vi "S4GUI_002.vi"(7 "Tab ObsEng":enum32{"Obs", "CCD modes", "Eng"}(tab)) -> ()   [LabVIEW 2018] (continued)
                      frame 0 {
                      }
                      frame 1 {
                      }
                      frame 2 {
                      }
                      frame 3 {
                        n288 = case shown="True" w572 {
                          tunnel: [cluster{u32, u32}[] [{7563008, 7563008}, {7563008, 7563008}] ("Colors [4]") cluster{u32, u32}[] [{16318208, 16318208}, {16318208, 16318208}] ("Colors [4]")] -> w571
                          frame False {
                          }
                          frame True {
                          }
                        }
                        n289 = Not(x=w572) -> (.not. x?=w573:bool)
                      }
                    }
                    "WPSEL Status" <- w554
                    "Waveplate" <- w554
                    n290 = property on="Waveplate" class="Bool (strict)"("Colors [4]"=w555, "BoolText.Text"=w551) -> ()  [unwired: 2 in, 2 out]
                    n291 = property on="WPSEL Status" class="Bool (strict)"("Colors [4]"=w555) -> ()  [unwired: 2 in, 2 out]
                  }
                  frame #1 {
                    # "WPROT"
                    n292 = Unbundle By Name(w579) -> ("WPROT State"=w578:i32)
                    n293 = case shown="2" w578 {
                      tunnel: [cluster{u32, u32}[] [{9868950, 9868950}, {9868950, 9868950}] ("Colors [4]") cluster{u32, u32}[] [{9868950, 9868950}, {9868950, 9868950}] ("Colors [4]") cluster{u32, u32}[] [{16318208, 16318208}, {16318208, 16318208}] ("Colors [4]") cluster{u32, u32}[] [{6618880, 6618880}, {6618880, 6618880}] ("Colors [4]") cluster{u32, u32}[] [{16318208, 16318208}, {16318208, 16318208}] ("Colors [4]")] -> w577
                      tunnel: [FALSE ("WPROT Status") FALSE ("WPROT Status") TRUE ("WPROT Status") FALSE ("WPROT Status") TRUE ("WPROT Status")] -> w576
                      frame Default {
                      }
                      frame 0 {
                      }
                      frame 1 {
                      }
                      frame 2 {
                      }
                      frame 3 {
                      }
                    }
                    "WPROT Status" <- w576
                    n294 = property on="WPROT Status" class="Bool (strict)"("Colors [4]"=w577) -> ()  [unwired: 2 in, 2 out]
                  }
                  frame #2 {
                    # "CALW"
                    n295 = Unbundle By Name(w597) -> ("CALW State"=w596:i32)
                    n296 = Unbundle By Name(w595) -> ("CALW posname"=w594:string)
                    n297 = local read "CALW Status"() -> (w590:bool)
                    n298 = case shown="3" w596 {
                      tunnel: [cluster{u32, u32}[] [{9868950, 9868950}, {9868950, 9868950}] ("Colors [4]") cluster{u32, u32}[] [{9868950, 9868950}, {9868950, 9868950}] ("Colors [4]") cluster{u32, u32}[] [{16318208, 16318208}, {16318208, 16318208}] ("Colors [4]") cluster{u32, u32}[] [{6618880, 6618880}, {6618880, 6618880}] ("Colors [4]") w617] -> w591
                      tunnel: [FALSE ("WPROT Status") FALSE ("WPROT Status") TRUE ("WPROT Status") FALSE ("WPROT Status") w619] -> w593
                      tunnel: w594 -> [_ _ _ w608 _]
                      tunnel: ["" "" "" w607 ""] -> w592
                      tunnel: w590 -> [_ _ _ _ w618]
                      frame Default {
                      }
                      frame 0 {
                      }
                      frame 1 {
                      }
                      frame 2 {
                        n299 = case shown="\"SHUTTER\"" w608 {
                          tunnel: ["" "DEPOL" "POL" "OFF" "PIN" "SHT"] -> w607
                          frame Default {
                          }
                          frame "DEPOLARIZER" {
                          }
                          frame "POLARIZER" {
                          }
                          frame "OFF" {
                          }
                          frame "PINHOLE" {
                          }
                          frame "SHUTTER" {
                          }
                        }
                      }
                      frame 3 {
                        n300 = case shown="False" w618 {
                          tunnel: [cluster{u32, u32}[] [{7563008, 7563008}, {7563008, 7563008}] ("Colors [4]") cluster{u32, u32}[] [{16318208, 16318208}, {16318208, 16318208}] ("Colors [4]")] -> w617
                          frame False {
                          }
                          frame True {
                          }
                        }
                        n301 = Not(x=w618) -> (.not. x?=w619:bool)
                      }
                    }
                    "CALW Status" <- w593
                    "PCS" <- w593
                    n302 = property on="CALW Status" class="Bool (strict)"("Colors [4]"=w591) -> ()  [unwired: 2 in, 2 out]
                    n303 = property on="PCS" class="Bool (strict)"("Colors [4]"=w591, "BoolText.Text"=w592) -> ()  [unwired: 2 in, 2 out]
                  }
                  frame #3 {
                    # "ASEL"
                    n304 = Unbundle By Name(w631) -> ("ASEL State"=w630:i32)
                    n305 = Unbundle By Name(w627) -> ("ASEL posname"=w624:string)
                    n306 = local read "ASEL Status"() -> (w625:bool)
                    n307 = case shown="Default" w624 {
                      selector: w624 -> [w632 _ _]
                      tunnel: [w632 "OFF" ("y") "ON" ("y")] -> w623
                      frame Default {
                      }
                      frame "OFF" {
                      }
                      frame "ON" {
                      }
                    }
                    n308 = case shown="3" w630 {
                      tunnel: [cluster{u32, u32}[] [{9868950, 9868950}, {9868950, 9868950}] ("Colors [4]") cluster{u32, u32}[] [{9868950, 9868950}, {9868950, 9868950}] ("Colors [4]") cluster{u32, u32}[] [{16318208, 16318208}, {16318208, 16318208}] ("Colors [4]") cluster{u32, u32}[] [{6618880, 6618880}, {6618880, 6618880}] ("Colors [4]") w650] -> w628
                      tunnel: [FALSE ("WPROT Status") FALSE ("WPROT Status") TRUE FALSE ("WPROT Status") w649] -> w629
                      tunnel: w623 -> [_ _ _ w645 _]
                      tunnel: ["" ("y") "" ("y") "" ("y") w645 "" ("y")] -> w626
                      tunnel: w625 -> [_ _ _ _ w647]
                      frame Default {
                      }
                      frame 0 {
                      }
                      frame 1 {
                      }
                      frame 2 {
                      }
                      frame 3 {
                        n309 = case shown="True" w647 {
                          tunnel: [cluster{u32, u32}[] [{7563008, 7563008}, {7563008, 7563008}] ("Colors [4]") cluster{u32, u32}[] [{16318208, 16318208}, {16318208, 16318208}] ("Colors [4]")] -> w650
                          frame False {
                          }
                          frame True {
                          }
                        }
                        n310 = Not(x=w647) -> (.not. x?=w649:bool)
                      }
                    }
                    "ASEL Status" <- w629
                    "Analyzer" <- w629
                    n311 = property on="Analyzer" class="Bool (strict)"("Colors [4]"=w628, "BoolText.Text"=w626) -> ()  [unwired: 2 in, 2 out]
                    n312 = property on="ASEL Status" class="Bool (strict)"("Colors [4]"=w628) -> ()  [unwired: 2 in, 2 out]
                  }
                  frame #4 {
                    # "GMIR & GFOC"
                    n313 = Unbundle By Name(w660) -> ("GMIR State"=w659:i32, "GFOC State"=w656:i32)
                    n314 = case shown="Default" w659 {
                      tunnel: [cluster{u32, u32}[] [{9868950, 9868950}, {9868950, 9868950}] ("Colors [4]") cluster{u32, u32}[] [{9868950, 9868950}, {9868950, 9868950}] ("Colors [4]") cluster{u32, u32}[] [{16318208, 16318208}, {16318208, 16318208}] ("Colors [4]") cluster{u32, u32}[] [{6618880, 6618880}, {6618880, 6618880}] ("Colors [4]") cluster{u32, u32}[] [{16318208, 16318208}, {16318208, 16318208}] ("Colors [4]")] -> w658
                      tunnel: [FALSE ("WPROT Status") FALSE ("WPROT Status") TRUE ("WPROT Status") FALSE ("WPROT Status") TRUE ("WPROT Status")] -> w655
                      frame Default {
                      }
                      frame 0 {
                      }
                      frame 1 {
                      }
                      frame 2 {
                      }
                      frame 3 {
                      }
                    }
                    "GMIR Status" <- w655
                    n315 = property on="GMIR Status" class="Bool (strict)"("Colors [4]"=w658) -> ()  [unwired: 2 in, 2 out]
                    n316 = case shown="Default" w656 {
                      tunnel: [cluster{u32, u32}[] [{9868950, 9868950}, {9868950, 9868950}] ("Colors [4]") cluster{u32, u32}[] [{9868950, 9868950}, {9868950, 9868950}] ("Colors [4]") cluster{u32, u32}[] [{16318208, 16318208}, {16318208, 16318208}] ("Colors [4]") cluster{u32, u32}[] [{6618880, 6618880}, {6618880, 6618880}] ("Colors [4]") cluster{u32, u32}[] [{16318208, 16318208}, {16318208, 16318208}] ("Colors [4]")] -> w657
                      tunnel: [FALSE ("WPROT Status") FALSE ("WPROT Status") TRUE ("WPROT Status") FALSE ("WPROT Status") TRUE ("WPROT Status")] -> w654
                      frame Default {
                      }
                      frame 0 {
                      }
                      frame 1 {
                      }
                      frame 2 {
                      }
                      frame 3 {
                      }
                    }
                    "GFOC Status" <- w654
                    n317 = Or(x=w655, y=w654) -> (x .or. y?=w653:bool)
                    n318 = property on="GFOC Status" class="Bool (strict)"("Colors [4]"=w657) -> ()  [unwired: 2 in, 2 out]
                    n319 = property on="GS led" class="Bool (strict)"("Blinking"=w653, "Value"=w653) -> ()  [unwired: 2 in, 2 out]
                  }
                }
              }
              frame #7 {
                n320 = Unbundle By Name(w683) -> ("Instrument Pos Names"=w682:T21)
                n321 = stacked-sequence {
                  tunnel: w682 -> [w685 w702 w727 w753]
                  tunnel: [_ _ _ w754] -> w681
                  frame #0 {
                    n322 = Unbundle By Name(w685) -> ("WPSEL posname"=w684:string)
                    n323 = case shown="\"L/2\", \"L/4\", \"OFF\"" w684 {
                      selector: w684 -> [_ w686]
                      frame "False", Default {
                      }
                      frame "L/2", "L/4", "OFF" {
                        n324 = First Call?() -> (First Call?: T/F=w687:bool)
                        n325 = case shown="True" w687 {
                          tunnel: w686 -> [_ w688]
                          frame False {
                          }
                          frame True {
                            n326 = case shown="\"OFF\"" w688 {
                              frame "False", Default {
                              }
                              frame "L/2" {
                                w689 = u16 1 items=["OFF", "Lambda/2", "Lambda/4"] ("Lambda Selector")
                                n327 = property on="Lambda Selector" class="Ring (strict)"(error in=errorcluster {"status"=FALSE, "code"=0, "source"=""} ("error in (no error)"), "Value"=w689) -> (error out=w691:errorcluster)  [unwired: 1 in, 1 out]
                                n328 = property on="Lambda Selector" class="Ring (strict)"(error in=w691, "RingText.Text"="Lambda/2" ("Boolean Text.Text")) -> ()  [unwired: 1 in, 2 out]
                              }
                              frame "L/4" {
                                w693 = u16 2 items=["OFF", "Lambda/2", "Lambda/4"] ("Lambda Selector")
                                n329 = property on="Lambda Selector" class="Ring (strict)"(error in=errorcluster {"status"=FALSE, "code"=0, "source"=""} ("error in (no error)"), "Value"=w693) -> (error out=w695:errorcluster)  [unwired: 1 in, 1 out]
                                n330 = property on="Lambda Selector" class="Ring (strict)"(error in=w695, "RingText.Text"="Lambda/4" ("Boolean Text.Text")) -> ()  [unwired: 1 in, 2 out]
                              }
                              frame "OFF" {
                                w698 = u16 0 items=["OFF", "Lambda/2", "Lambda/4"] ("Lambda Selector")
                                (unwired) "Select..." ("Boolean Text.Text")
                                n331 = property on="Lambda Selector" class="Ring (strict)"(error in=errorcluster {"status"=FALSE, "code"=0, "source"=""} ("error in (no error)"), "Value"=w698) -> (error out=w700:errorcluster)  [unwired: 1 in, 1 out]
                                n332 = property on="Lambda Selector" class="Ring (strict)"(error in=w700, "RingText.Text"="OFF" ("Boolean Text.Text")) -> ()  [unwired: 1 in, 2 out]
                              }
                            }
                          }
                        }
                      }
                    }
                  }
                  frame #1 {
                    n333 = Unbundle By Name(w702) -> ("CALW posname"=w701:string)
                    n334 = case shown="\"DEPOLARIZER\", \"OFF\", \"PINHOLE\", \"POLARIZER\", \"SHUTTER\"" w701 {
                      selector: w701 -> [_ w703]
                      frame "False", Default {
                      }
                      frame "DEPOLARIZER", "OFF", "PINHOLE", "POLARIZER", "SHUTTER" {
                        n335 = First Call?() -> (First Call?: T/F=w704:bool)
                        n336 = case shown="True" w704 {
                          tunnel: w703 -> [_ w705]
                          frame False {
                          }
                          frame True {
                            n337 = case shown="\"OFF\"" w705 {
                              frame "False", Default {
                              }
                              frame "POLARIZER" {
                                w706 = u16 1 items=["OFF", "POLARIZER", "PINHOLE", "SHUTTER", "DEPOLARIZER"] ("Calibrator Selector")
                                n338 = property on="Calibrator Selector" class="Ring (strict)"(error in=errorcluster {"status"=FALSE, "code"=0, "source"=""} ("error in (no error)"), "Value"=w706) -> (error out=w708:errorcluster)  [unwired: 1 in, 1 out]
                                n339 = property on="Calibrator Selector" class="Ring (strict)"(error in=w708, "RingText.Text"="POLARIZER" ("Boolean Text.Text")) -> ()  [unwired: 1 in, 2 out]
                              }
                              frame "DEPOLARIZER" {
                                w710 = u16 4 items=["OFF", "POLARIZER", "PINHOLE", "SHUTTER", "DEPOLARIZER"] ("Calibrator Selector")
                                n340 = property on="Calibrator Selector" class="Ring (strict)"(error in=errorcluster {"status"=FALSE, "code"=0, "source"=""} ("error in (no error)"), "Value"=w710) -> (error out=w712:errorcluster)  [unwired: 1 in, 1 out]
                                n341 = property on="Calibrator Selector" class="Ring (strict)"(error in=w712, "RingText.Text"="DEPOLARIZER" ("Boolean Text.Text")) -> ()  [unwired: 1 in, 2 out]
                              }
                              frame "PINHOLE" {
                                w714 = u16 2 items=["OFF", "POLARIZER", "PINHOLE", "SHUTTER", "DEPOLARIZER"] ("Calibrator Selector")
                                n342 = property on="Calibrator Selector" class="Ring (strict)"(error in=errorcluster {"status"=FALSE, "code"=0, "source"=""} ("error in (no error)"), "Value"=w714) -> (error out=w716:errorcluster)  [unwired: 1 in, 1 out]
                                n343 = property on="Calibrator Selector" class="Ring (strict)"(error in=w716, "RingText.Text"="PINHOLE" ("Boolean Text.Text")) -> ()  [unwired: 1 in, 2 out]
                              }
                              frame "SHUTTER" {
                                w718 = u16 3 items=["OFF", "POLARIZER", "PINHOLE", "SHUTTER", "DEPOLARIZER"] ("Calibrator Selector")
                                n344 = property on="Calibrator Selector" class="Ring (strict)"(error in=errorcluster {"status"=FALSE, "code"=0, "source"=""} ("error in (no error)"), "Value"=w718) -> (error out=w720:errorcluster)  [unwired: 1 in, 1 out]
                                n345 = property on="Calibrator Selector" class="Ring (strict)"(error in=w720, "RingText.Text"="SHUTTER" ("Boolean Text.Text")) -> ()  [unwired: 1 in, 2 out]
                              }
                              frame "OFF" {
                                w722 = u16 0 items=["OFF", "POLARIZER", "PINHOLE", "SHUTTER", "DEPOLARIZER"] ("Calibrator Selector")
                                n346 = property on="Calibrator Selector" class="Ring (strict)"(error in=errorcluster {"status"=FALSE, "code"=0, "source"=""} ("error in (no error)"), "Value"=w722) -> (error out=w724:errorcluster)  [unwired: 1 in, 1 out]
                                n347 = property on="Calibrator Selector" class="Ring (strict)"(error in=w724, "RingText.Text"="OFF" ("Boolean Text.Text")) -> ()  [unwired: 1 in, 2 out]
                              }
                            }
                          }
                        }
                      }
                    }
                  }
                  frame #2 {
                    n348 = Unbundle By Name(w727) -> ("WPROT posname"=w726:string)
                    "Name" <- w726
                    n349 = stacked-sequence {
                      tunnel: w726 -> [_ w729]
                      frame #0 {
                        w728 = FALSE
                        "ledP0" <- w728
                        "ledP1" <- w728
                        "ledP2" <- w728
                        "ledP3" <- w728
                        "ledP4" <- w728
                        "ledP5" <- w728
                        "ledP6" <- w728
                        "ledP7" <- w728
                        "ledP8" <- w728
                        "ledP9" <- w728
                        "ledP10" <- w728
                        "ledP11" <- w728
                        "ledP12" <- w728
                        "ledP13" <- w728
                        "ledP14" <- w728
                        "ledP15" <- w728
                      }
                      frame #1 {
                        n350 = case shown="\"WP3\"" w729 {
                          frame Default {
                          }
                          frame "WP1" {
                            n351 = local write "ledP0"(TRUE ("ledP0")) -> ()
                          }
                          frame "WP2" {
                            n352 = local write "ledP1"(TRUE ("ledP0")) -> ()
                          }
                          frame "WP3" {
                            n353 = local write "ledP2"(TRUE ("ledP0")) -> ()
                          }
                          frame "WP4" {
                            n354 = local write "ledP3"(TRUE ("ledP0")) -> ()
                          }
                          frame "WP5" {
                            n355 = local write "ledP4"(TRUE ("ledP0")) -> ()
                          }
                          frame "WP6" {
                            n356 = local write "ledP5"(TRUE ("ledP0")) -> ()
                          }
                          frame "WP7" {
                            n357 = local write "ledP6"(TRUE ("ledP0")) -> ()
                          }
                          frame "WP8" {
                            n358 = local write "ledP7"(TRUE ("ledP0")) -> ()
                          }
                          frame "WP9" {
                            n359 = local write "ledP8"(TRUE ("ledP0")) -> ()
                          }
                          frame "WP10" {
                            n360 = local write "ledP9"(TRUE ("ledP0")) -> ()
                          }
                          frame "WP11" {
                            n361 = local write "ledP10"(TRUE ("ledP0")) -> ()
                          }
                          frame "WP12" {
                            n362 = local write "ledP11"(TRUE ("ledP0")) -> ()
                          }
                          frame "WP13" {
                            n363 = local write "ledP12"(TRUE ("ledP0")) -> ()
                          }
                          frame "WP14" {
                            n364 = local write "ledP13"(TRUE ("ledP0")) -> ()
                          }
                          frame "WP15" {
                            n365 = local write "ledP14"(TRUE ("ledP0")) -> ()
                          }
                          frame "WP16" {
                            n366 = local write "ledP15"(TRUE ("ledP0")) -> ()
                          }
                        }
                      }
                    }
                  }
                  frame #3 {
                    w757 = "OFF" ("Boolean Text.Text")
                    # "Polarimetria:   ASEL = ON  &   (WPSEL =L/2 or L/4)\n\nFotometria:    ASEL=OFF & WPSEL = OFF & CALW = OFF"
                    n367 = Unbundle By Name(w753) -> ("ASEL posname"=w748:string, "WPSEL posname"=w750:string, "CALW posname"=w749:string)
                    n368 = Unbundle By Name(w753) -> ("WPSEL posname"=w760:string, "CALW posname"=w761:string, "ASEL posname"=w755:string)
                    n369 = Equal?(x=w748, y="ON" ("Boolean Text.Text")) -> (x = y?=w751:bool)
                    n370 = case shown="True" w751 {
                      tunnel: w750 -> [w770 w779]
                      tunnel: w749 -> [w769 w773]
                      tunnel: w748 -> [w766 _]
                      tunnel: [FALSE ("Polarimetric Mode") w774] -> w747
                      tunnel: [w762 FALSE ("Photometric Mode")] -> w746
                      frame False {
                        w765 = "OFF" ("Boolean Text.Text")
                        n371 = Equal?(x=w766, y=w765) -> (x = y?=w764:bool)
                        n372 = Equal?(x=w769, y=w765) -> (x = y?=w767:bool)
                        n373 = Equal?(x=w770, y=w765) -> (x = y?=w768:bool)
                        n374 = Compound Arithmetic op=AND(w764, w768, w767) -> (w762:bool)
                      }
                      frame True {
                        n375 = Equal?(x="L/2" ("Boolean Text.Text"), y=w779) -> (x = y?=w780:bool)
                        n376 = Equal?(x="L/4" ("Boolean Text.Text"), y=w779) -> (x = y?=w777:bool)
                        n377 = Not Equal?(x="SHUTTER", y=w773) -> (x != y?=w771:bool)
                        n378 = Or(x=w780, y=w777) -> (x .or. y?=w775:bool)
                        n379 = And(x=w775, y=w771) -> (x .and. y?=w774:bool)
                      }
                    }
                    "Polarimetric Mode" <- w747
                    "Photometric Mode" <- w746
                    n380 = Equal?(x=w757, y=w760) -> (x = y?=w758:bool)
                    n381 = Equal?(x=w757, y=w761) -> (x = y?=w759:bool)
                    n382 = Equal?(x=w757, y=w755) -> (x = y?=w756:bool)
                    n383 = Compound Arithmetic op=AND(w758, w759, w756) -> (invert w754:bool)
                  }
                }
              }
              frame #8 {
                n384 = Unbundle By Name(w786) -> ("ChannelA_Status"=w785:T22, "ChannelB_Status"=w784:T22, "ChannelC_Status"=w782:T22, "ChannelD_Status"=w783:T22)
                n385 = stacked-sequence {
                  tunnel: w785 -> [w874 w930 w982 w1059 _ _ _]
                  tunnel: w784 -> [w873 w928 w981 _ w1080 _ _]
                  tunnel: w783 -> [w871 w925 w979 _ _ _ w1122]
                  tunnel: w782 -> [w872 w926 w980 _ _ w1101 _]
                  frame #0 {
                    n386 = Unbundle By Name(w871) -> ("connection"=w851:bool, "FT"=w833:bool, "Current exp"=w810:dbl, "Cooler ON/OFF"=w865:i16, "Currently temperature"=w862:i16, "Temperature Status"=w859:string, "target  temp"=w795:i16)
                    "Exposure Time ch4" <- w810
                    n387 = Unbundle By Name(w873) -> ("connection"=w853:bool, "FT"=w837:bool, "Current exp"=w821:dbl, "Cooler ON/OFF"=w867:i16, "Currently temperature"=w864:i16, "Temperature Status"=w861:string, "target  temp"=w799:i16)
                    "Exposure Time ch2" <- w821
                    n388 = Unbundle By Name(w874) -> ("connection"=w854:bool, "FT"=w838:bool, "Current exp"=w830:dbl, "Cooler ON/OFF"=w870:i16, "Currently temperature"=w868:i16, "Temperature Status"=w869:string, "target  temp"=w807:i16)
                    "Exposure Time ch1" <- w830
                    n389 = Unbundle By Name(w872) -> ("connection"=w852:bool, "FT"=w835:bool, "Current exp"=w811:dbl, "Cooler ON/OFF"=w866:i16, "Currently temperature"=w863:i16, "Temperature Status"=w860:string, "target  temp"=w796:i16)
                    "Exposure Time ch3" <- w811
                    n390 = Number To Decimal String(number=w795) -> (decimal integer string=→"Target Temp 4":string)  [unwired: 1 in]
                    n391 = Number To Decimal String(number=w796) -> (decimal integer string=→"Target Temp 3":string)  [unwired: 1 in]
                    n392 = Number To Decimal String(number=w799) -> (decimal integer string=→"Target Temp 2":string)  [unwired: 1 in]
                    n393 = Not Equal To 0?(x=w865) -> (x != 0?=w856:bool)
                    n394 = First Call?() -> (First Call?: T/F=w848:bool)
                    n395 = First Call?() -> (First Call?: T/F=w850:bool)
                    n396 = First Call?() -> (First Call?: T/F=w847:bool)
                    n397 = Not Equal To 0?(x=w866) -> (x != 0?=w855:bool)
                    n398 = First Call?() -> (First Call?: T/F=w849:bool)
                    n399 = Number To Decimal String(number=w807) -> (decimal integer string=→"Target Temp 1":string)  [unwired: 1 in]
                    n400 = Number To Fractional String(use system decimal point (T)=FALSE, number=w830, precision (6)=i16 2) -> (F-format string=w827:string)  [unwired: 1 in]
                    n401 = case shown="True" w848 {
                      tunnel: w796 -> [_ w876]
                      frame False {
                      }
                      frame True {
                        n402 = property on="Target Temp 3" class="DigNum (strict)"("Value"=w876) -> ()  [unwired: 2 in, 2 out]
                      }
                    }
                    n403 = case shown="True" w850 {
                      tunnel: w807 -> [_ w878]
                      frame False {
                      }
                      frame True {
                        n404 = property on="Target Temp 1" class="DigNum (strict)"("Value"=w878) -> ()  [unwired: 2 in, 2 out]
                      }
                    }
                    n405 = Number To Fractional String(use system decimal point (T)=FALSE, number=w821, precision (6)=i16 2) -> (F-format string=w822:string)  [unwired: 1 in]
                    n406 = case shown="True" w847 {
                      tunnel: w795 -> [_ w875]
                      frame False {
                      }
                      frame True {
                        n407 = property on="Target Temp 4" class="DigNum (strict)"("Value"=w875) -> ()  [unwired: 2 in, 2 out]
                      }
                    }
                    n408 = Concatenate Strings("Exposure Time ", w827) -> (w826:string)
                    n409 = Number To Fractional String(use system decimal point (T)=FALSE, number=w811, precision (6)=i16 2) -> (F-format string=w812:string)  [unwired: 1 in]
                    n410 = Number To Fractional String(use system decimal point (T)=FALSE, number=w810, precision (6)=i16 2) -> (F-format string=w816:string)  [unwired: 1 in]
                    n411 = Concatenate Strings("Exposure Time ", w822) -> (w820:string)
                    n412 = case shown="True" w849 {
                      tunnel: w799 -> [_ w877]
                      frame False {
                      }
                      frame True {
                        n413 = property on="Target Temp 2" class="DigNum (strict)"("Value"=w877) -> ()  [unwired: 2 in, 2 out]
                      }
                    }
                    n414 = Concatenate Strings("Exposure Time ", w812) -> (w808:string)
                    n415 = Concatenate Strings("Exposure Time ", w816) -> (w809:string)
                    n416 = property on="Exposure Time ch1" class="Slide (strict)"("Caption.Text"=w826) -> ()  [unwired: 2 in, 2 out]
                    n417 = property on="Exposure Time ch2" class="Slide (strict)"("Caption.Text"=w820) -> ()  [unwired: 2 in, 2 out]
                    n418 = property on="Exposure Time ch3" class="Slide (strict)"("Caption.Text"=w808) -> ()  [unwired: 2 in, 2 out]
                    n419 = property on="Exposure Time ch4" class="Slide (strict)"("Caption.Text"=w809) -> ()  [unwired: 2 in, 2 out]
                    n420 = Not Equal To 0?(x=w870) -> (x != 0?=w857:bool)
                    n421 = Not Equal To 0?(x=w867) -> (x != 0?=w858:bool)
                    n422 = case shown="True" w854 {
                      tunnel: w869 -> [_ w909]
                      tunnel: w868 -> [_ w910]
                      tunnel: w857 -> [_ w907]
                      tunnel: [FALSE w907] -> w846
                      tunnel: [i16 0 ("Currently temperature") w910] -> w804
                      tunnel: ["" ("Temperature Status") w909] -> w845
                      tunnel: [FALSE w908] -> w839
                      tunnel: w838 -> [_ w908]
                      frame False {
                      }
                      frame True {
                      }
                    }
                    "Cooler status 1" <- w846
                    "Curr Temp 1" <- w804
                    "Temp Status 1" <- w845
                    "Panel Temp" <- w804
                    "Panel cooler 1" <- w846
                    "FT1" <- w839
                    n423 = case shown="False" w853 {
                      tunnel: w864 -> [_ w901]
                      tunnel: w861 -> [_ w900]
                      tunnel: w858 -> [_ w902]
                      tunnel: [FALSE w902] -> w844
                      tunnel: [i16 0 ("Currently temperature") w901] -> w800
                      tunnel: ["" ("Temperature Status") w900] -> w843
                      tunnel: w837 -> [_ w899]
                      tunnel: [FALSE ("FT") w899] -> w836
                      frame False {
                      }
                      frame True {
                      }
                    }
                    "Panel Temp 2" <- w800
                    "Curr Temp 2" <- w800
                    "Cooler status 2" <- w844
                    "Panel cooler 2" <- w844
                    "Temp Status 2" <- w843
                    "FT2" <- w836
                    n424 = case shown="True" w851 {
                      tunnel: w862 -> [_ w885]
                      tunnel: w859 -> [_ w884]
                      tunnel: w856 -> [_ w886]
                      tunnel: [FALSE w886] -> w841
                      tunnel: [i16 0 ("Currently temperature") w885] -> w788
                      tunnel: ["" ("Temperature Status") w884] -> w840
                      tunnel: w833 -> [_ w883]
                      tunnel: [FALSE ("FT") w883] -> w832
                      frame False {
                      }
                      frame True {
                      }
                    }
                    "Cooler status 4" <- w841
                    "Panel Temp 4" <- w788
                    "Curr Temp 4" <- w788
                    "Temp Status 4" <- w840
                    "Panel cooler 4" <- w841
                    "FT4" <- w832
                    n425 = case shown="True" w852 {
                      tunnel: w863 -> [_ w893]
                      tunnel: w860 -> [_ w892]
                      tunnel: w855 -> [_ w894]
                      tunnel: [FALSE w894] -> w842
                      tunnel: [i16 0 ("Currently temperature") w893] -> w789
                      tunnel: ["" ("Temperature Status") w892] -> w787
                      tunnel: w835 -> [_ w891]
                      tunnel: [FALSE ("FT") w891] -> w834
                      frame False {
                      }
                      frame True {
                      }
                    }
                    "Cooler status 3" <- w842
                    "Panel Temp 3" <- w789
                    "Curr Temp 3" <- w789
                    "Panel cooler 3" <- w842
                    "FT3" <- w834
                    "Temp Status 3" <- w787
                    n426 = Number To Decimal String(number=w800) -> (decimal integer string=w801:string)  [unwired: 1 in]
                    n427 = Number To Decimal String(number=w804) -> (decimal integer string=w805:string)  [unwired: 1 in]
                    n428 = property on="Panel cooler 2" class="Bool (strict)"("BoolText.Text"=w801, "BoolText.Justify"=enum16{"Left", "Center", "Right"}."Right" ("Boolean Text.Justification")) -> ()  [unwired: 2 in, 2 out]
                    n429 = property on="Panel cooler 1" class="Bool (strict)"("BoolText.Text"=w805, "BoolText.Justify"=enum16{"Left", "Center", "Right"}."Right" ("Boolean Text.Justification")) -> ()  [unwired: 2 in, 2 out]
                    n430 = Number To Decimal String(number=w789) -> (decimal integer string=w793:string)  [unwired: 1 in]
                    n431 = Number To Decimal String(number=w788) -> (decimal integer string=w790:string)  [unwired: 1 in]
                    n432 = property on="Panel cooler 3" class="Bool (strict)"("BoolText.Text"=w793, "BoolText.Justify"=enum16{"Left", "Center", "Right"}."Right" ("Boolean Text.Justification")) -> ()  [unwired: 2 in, 2 out]
                    n433 = property on="Panel cooler 4" class="Bool (strict)"("BoolText.Text"=w790, "BoolText.Justify"=enum16{"Left", "Center", "Right"}."Right" ("Boolean Text.Justification")) -> ()  [unwired: 2 in, 2 out]
                  }
                  frame #1 {
                    n434 = Unbundle By Name(w925) -> ("LastFileImage"=→"Last Image ch4":string, "Temperature Status"=w913:string)
                    n435 = Unbundle By Name(w926) -> ("LastFileImage"=→"Last Image ch3":string, "Temperature Status"=w914:string)
                    n436 = Unbundle By Name(w928) -> ("LastFileImage"=→"Last Image ch2":string, "Temperature Status"=w917:string)
                    n437 = Unbundle By Name(w930) -> ("LastFileImage"=→"Last Image ch1":string, "Temperature Status"=w922:string)
                    n438 = case shown="Default" w922 {
                      tunnel: [cluster{u32, u32}[] [{6124107, 6124107}, {6124107, 6124107}] ("Colors [4]") cluster{u32, u32}[] [{6618880, 6618880}, {6618880, 6618880}] ("Colors [4]") cluster{u32, u32}[] [{16318208, 16318208}, {16318208, 16318208}] ("Colors [4]") cluster{u32, u32}[] [{8554752, 8554752}, {8554752, 8554752}] ("Colors [4]")] -> w921
                      tunnel: [FALSE FALSE FALSE TRUE] -> w920
                      frame Default {
                      }
                      frame "TEMPERATURE_STABILIZED" {
                      }
                      frame "TEMPERATURE_NOT_STABILIZED" {
                      }
                      frame "TEMPERATURE_NOT_REACHED" {
                      }
                    }
                    n439 = case shown="\"TEMPERATURE_NOT_REACHED\"" w917 {
                      tunnel: [cluster{u32, u32}[] [{6124107, 6124107}, {6124107, 6124107}] ("Colors [4]") cluster{u32, u32}[] [{6618880, 6618880}, {6618880, 6618880}] ("Colors [4]") cluster{u32, u32}[] [{16318208, 16318208}, {16318208, 16318208}] ("Colors [4]") cluster{u32, u32}[] [{8554752, 8554752}, {8554752, 8554752}] ("Colors [4]")] -> w919
                      tunnel: [FALSE FALSE FALSE TRUE] -> w918
                      frame Default {
                      }
                      frame "TEMPERATURE_STABILIZED" {
                      }
                      frame "TEMPERATURE_NOT_STABILIZED" {
                      }
                      frame "TEMPERATURE_NOT_REACHED" {
                      }
                    }
                    n440 = case shown="\"TEMPERATURE_NOT_REACHED\"" w914 {
                      tunnel: [cluster{u32, u32}[] [{6124107, 6124107}, {6124107, 6124107}] ("Colors [4]") cluster{u32, u32}[] [{6618880, 6618880}, {6618880, 6618880}] ("Colors [4]") cluster{u32, u32}[] [{16318208, 16318208}, {16318208, 16318208}] ("Colors [4]") cluster{u32, u32}[] [{8554752, 8554752}, {8554752, 8554752}] ("Colors [4]")] -> w916
                      tunnel: [FALSE FALSE FALSE TRUE] -> w915
                      frame Default {
                      }
                      frame "TEMPERATURE_STABILIZED" {
                      }
                      frame "TEMPERATURE_NOT_STABILIZED" {
                      }
                      frame "TEMPERATURE_NOT_REACHED" {
                      }
                    }
                    n441 = case shown="\"TEMPERATURE_NOT_REACHED\"" w913 {
                      tunnel: [cluster{u32, u32}[] [{6124107, 6124107}, {6124107, 6124107}] ("Colors [4]") cluster{u32, u32}[] [{6618880, 6618880}, {6618880, 6618880}] ("Colors [4]") cluster{u32, u32}[] [{16318208, 16318208}, {16318208, 16318208}] ("Colors [4]") cluster{u32, u32}[] [{8554752, 8554752}, {8554752, 8554752}] ("Colors [4]")] -> w912
                      tunnel: [FALSE FALSE FALSE TRUE] -> w911
                      frame Default {
                      }
                      frame "TEMPERATURE_STABILIZED" {
                      }
                      frame "TEMPERATURE_NOT_STABILIZED" {
                      }
                      frame "TEMPERATURE_NOT_REACHED" {
                      }
                    }
                    n442 = property on="Cooler status 1" class="Bool (strict)"("Colors [4]"=w921, "Blinking"=w920) -> ()  [unwired: 2 in, 2 out]
                    n443 = property on="Panel cooler 1" class="Bool (strict)"("Colors [4]"=w921, "Blinking"=w920) -> ()  [unwired: 2 in, 2 out]
                    n444 = property on="Cooler status 4" class="Bool (strict)"("Colors [4]"=w912, "Blinking"=w911) -> ()  [unwired: 2 in, 2 out]
                    n445 = property on="Cooler status 3" class="Bool (strict)"("Colors [4]"=w916, "Blinking"=w915) -> ()  [unwired: 2 in, 2 out]
                    n446 = property on="Panel cooler 4" class="Bool (strict)"("Colors [4]"=w912, "Blinking"=w911) -> ()  [unwired: 2 in, 2 out]
                    n447 = property on="Cooler status 2" class="Bool (strict)"("Colors [4]"=w919, "Blinking"=w918) -> ()  [unwired: 2 in, 2 out]
                    n448 = property on="Panel cooler 3" class="Bool (strict)"("Colors [4]"=w916, "Blinking"=w915) -> ()  [unwired: 2 in, 2 out]
                    n449 = property on="Panel cooler 2" class="Bool (strict)"("Colors [4]"=w919, "Blinking"=w918) -> ()  [unwired: 2 in, 2 out]
                  }
                  frame #2 {
                    n450 = Unbundle By Name(w981) -> ("CamStatus"=w974:string, "connection"=w973:bool)
                    n451 = Unbundle By Name(w980) -> ("CamStatus"=w970:string, "connection"=w969:bool)
                    n452 = Unbundle By Name(w979) -> ("CamStatus"=w966:string, "connection"=w965:bool)
                    n453 = Unbundle By Name(w982) -> ("CamStatus"=w978:string, "connection"=w976:bool)
                    n454 = case shown="True" w973 {
                      tunnel: w974 -> [_ w1013]
                      tunnel: [u32 16739417 w1014] -> w971
                      tunnel: ["" ("CamStatus") w1013] -> w972
                      frame False {
                      }
                      frame True {
                        n455 = property on="Acq status string ch2" class="Str"() -> ("Text.BGColor"=w1015:u32)  [unwired: 2 in, 2 out]
                        n456 = case shown="\"\"" w1013 {
                          tunnel: [u32 16688641 w1020 u32 13882323 u32 13882323] -> w1014
                          tunnel: w1015 -> [_ w1019 _ _]
                          frame Default {
                            # "WAITING_EXPOSE_COMMAND"
                          }
                          frame "ACTIVE" {
                            n457 = Equal?(x=w1019, y=u32 16776002) -> (x = y?=w1018:bool)
                            n458 = case shown="False" w1018 {
                              tunnel: [u32 16776002 u32 16449369] -> w1020
                              frame False {
                              }
                              frame True {
                              }
                            }
                          }
                          frame "IDLE" {
                          }
                          frame "" {
                            # "sem resposta do ACS"
                          }
                        }
                      }
                    }
                    "Acq status string ch2" <- w972
                    n459 = case shown="True" w965 {
                      tunnel: w966 -> [_ w985]
                      tunnel: [u32 16739417 w986] -> w963
                      tunnel: ["" ("CamStatus") w985] -> w964
                      frame False {
                      }
                      frame True {
                        n460 = property on="Acq status string ch4" class="Str"() -> ("Text.BGColor"=w987:u32)  [unwired: 2 in, 2 out]
                        n461 = case shown="\"IDLE\"" w985 {
                          tunnel: [u32 16688641 w992 u32 13882323 u32 13882323] -> w986
                          tunnel: w987 -> [_ w991 _ _]
                          frame Default {
                            # "WAITING_EXPOSE_COMMAND"
                          }
                          frame "ACTIVE" {
                            n462 = Equal?(x=w991, y=u32 16776002) -> (x = y?=w990:bool)
                            n463 = case shown="False" w990 {
                              tunnel: [u32 16776002 u32 16449369] -> w992
                              frame False {
                              }
                              frame True {
                              }
                            }
                          }
                          frame "IDLE" {
                          }
                          frame "" {
                            # "sem resposta do ACS"
                          }
                        }
                      }
                    }
                    "Acq status string ch4" <- w964
                    n464 = case shown="True" w969 {
                      tunnel: w970 -> [_ w999]
                      tunnel: [u32 16739417 w1000] -> w967
                      tunnel: ["" ("CamStatus") w999] -> w968
                      frame False {
                      }
                      frame True {
                        n465 = property on="Acq status string ch3" class="Str"() -> ("Text.BGColor"=w1001:u32)  [unwired: 2 in, 2 out]
                        n466 = case shown="\"\"" w999 {
                          tunnel: [u32 16688641 w1006 u32 13882323 u32 13882323] -> w1000
                          tunnel: w1001 -> [_ w1005 _ _]
                          frame Default {
                            # "WAITING_EXPOSE_COMMAND"
                          }
                          frame "ACTIVE" {
                            n467 = Equal?(x=w1005, y=u32 16776002) -> (x = y?=w1004:bool)
                            n468 = case shown="False" w1004 {
                              tunnel: [u32 16776002 u32 16449369] -> w1006
                              frame False {
                              }
                              frame True {
                              }
                            }
                          }
                          frame "IDLE" {
                          }
                          frame "" {
                            # "sem resposta do ACS"
                          }
                        }
                      }
                    }
                    "Acq status string ch3" <- w968
                    n469 = case shown="True" w976 {
                      tunnel: w978 -> [_ w1027]
                      tunnel: [u32 16739417 w1028] -> w977
                      tunnel: ["" ("CamStatus") w1027] -> w975
                      frame False {
                      }
                      frame True {
                        n470 = property on="Acq status string ch1" class="Str"() -> ("Text.BGColor"=w1029:u32)  [unwired: 2 in, 2 out]
                        n471 = case shown="\"\"" w1027 {
                          tunnel: [u32 16688641 w1034 u32 13882323 u32 13882323] -> w1028
                          tunnel: w1029 -> [_ w1033 _ _]
                          frame Default {
                            # "WAITING_EXPOSE_COMMAND"
                          }
                          frame "ACTIVE" {
                            n472 = Equal?(x=w1033, y=u32 16776002) -> (x = y?=w1032:bool)
                            n473 = case shown="False" w1032 {
                              tunnel: [u32 16776002 u32 16449369] -> w1034
                              frame False {
                              }
                              frame True {
                              }
                            }
                          }
                          frame "IDLE" {
                          }
                          frame "" {
                            # "sem resposta do ACS"
                          }
                        }
                      }
                    }
                    "Acq status string ch1" <- w975
                    n474 = property on="Acq status string ch2" class="Str"("Text.BGColor"=w971) -> ()  [unwired: 2 in, 2 out]
                    n475 = property on="Acq status string ch1" class="Str"("Text.BGColor"=w977) -> ()  [unwired: 2 in, 2 out]
                    n476 = property on="Acq status string ch3" class="Str"("Text.BGColor"=w967) -> ()  [unwired: 2 in, 2 out]
                    n477 = property on="Acq status string ch4" class="Str"("Text.BGColor"=w963) -> ()  [unwired: 2 in, 2 out]
                  }
                  frame #3 {
                    w1047 = cluster{u32, u32}[] [{16711680, 16711680}, {15400704, 15400704}, {16776722, 0}, {16776722, 0}]  # amarelo
                    w1046 = cluster{u32, u32}[] [{16711680, 16711680}, {6618880, 6618880}, {16776722, 0}, {16776722, 0}]  # verde
                    # "Se ocupacao do disco maior que\n90%, barra em vermelho."
                    # "Atualiza status CANAL 1"
                    n478 = Unbundle By Name(w1059) -> ("Frames done"=w1056:u32, "connection"=→"Channel 1" →"setupCH1":bool, "conf runing"=w1057:bool, "UsedDisk"=w1041:u16, "operational"=w1044:bool)
                    "Exposures Done ch1" <- w1056
                    "Disk Storage ch1" <- w1041
                    n479 = Number To Decimal String(number=w1056) -> (decimal integer string=w1054:string)  [unwired: 1 in]
                    n480 = Greater?(x=w1041, y=u16 90) -> (0:w1051:bool)
                    n481 = Select(t=u32 16711680, s=w1051, f=u32 16860) -> (s? t:f=w1049:u32)
                    n482 = Concatenate Strings("#Exposures Done ", w1054) -> (w1053:string)
                    n483 = Select(t=w1046, s=w1044, f=w1047) -> (s? t:f=w1045:cluster{u32, u32}[])
                    n484 = property on="setupCH1" class="Bool (strict)"("Blinking"=w1057) -> ()  [unwired: 2 in, 2 out]
                    n485 = property on="Exposures Done ch1" class="Slide (strict)"("Caption.Text"=w1053) -> ()  [unwired: 2 in, 2 out]
                    n486 = property on="Channel 1" class="Bool (strict)"("Colors [4]"=w1045) -> ()  [unwired: 2 in, 2 out]
                    n487 = property on="Disk Storage ch1" class="Slide (strict)"("Fill Color"=w1049) -> ()  [unwired: 2 in, 2 out]
                    n488 = Number To Decimal String(number=w1041) -> (decimal integer string=w1042:string)  [unwired: 1 in]
                    n489 = Concatenate Strings("Disk Storage ", w1042, "%" ("string")) -> (w1040:string)
                    n490 = property on="Disk Storage ch1" class="Slide (strict)"("Caption.Text"=w1040) -> ()  [unwired: 2 in, 2 out]
                  }
                  frame #4 {
                    w1068 = cluster{u32, u32}[] [{16711680, 16711680}, {15400704, 15400704}, {16776722, 0}, {16776722, 0}]  # amarelo
                    w1067 = cluster{u32, u32}[] [{16711680, 16711680}, {6618880, 6618880}, {16776722, 0}, {16776722, 0}]  # verde
                    # "Se ocupacao do disco maior que\n90%, barra em vermelho."
                    # "Atualiza status CANAL 2"
                    n491 = Unbundle By Name(w1080) -> ("Frames done"=w1075:u32, "connection"=→"Channel 2" →"setupCH2":bool, "conf runing"=w1078:bool, "UsedDisk"=w1060:u16, "operational"=w1065:bool)
                    "Exposures Done ch2" <- w1075
                    "Disk Storage ch2" <- w1060
                    n492 = Number To Decimal String(number=w1075) -> (decimal integer string=w1076:string)  [unwired: 1 in]
                    n493 = Greater?(x=w1060, y=u16 90) -> (0:w1072:bool)
                    n494 = Select(t=u32 16711680, s=w1072, f=u32 16860) -> (s? t:f=w1069:u32)
                    n495 = Concatenate Strings("#Exposures Done ", w1076) -> (w1074:string)
                    n496 = Select(t=w1067, s=w1065, f=w1068) -> (s? t:f=w1066:cluster{u32, u32}[])
                    n497 = property on="setupCH2" class="Bool (strict)"("Blinking"=w1078) -> ()  [unwired: 2 in, 2 out]
                    n498 = property on="Disk Storage ch2" class="Slide (strict)"("Fill Color"=w1069) -> ()  [unwired: 2 in, 2 out]
                    n499 = property on="Exposures Done ch2" class="Slide (strict)"("Caption.Text"=w1074) -> ()  [unwired: 2 in, 2 out]
                    n500 = property on="Channel 2" class="Bool (strict)"("Colors [4]"=w1066) -> ()  [unwired: 2 in, 2 out]
                    n501 = Number To Decimal String(number=w1060) -> (decimal integer string=w1063:string)  [unwired: 1 in]
                    n502 = Concatenate Strings("Disk Storage ", w1063, "%" ("string")) -> (w1061:string)
                    n503 = property on="Disk Storage ch2" class="Slide (strict)"("Caption.Text"=w1061) -> ()  [unwired: 2 in, 2 out]
                  }
                  frame #5 {
                    w1089 = cluster{u32, u32}[] [{16711680, 16711680}, {15400704, 15400704}, {16776722, 0}, {16776722, 0}]  # amarelo
                    w1088 = cluster{u32, u32}[] [{16711680, 16711680}, {6618880, 6618880}, {16776722, 0}, {16776722, 0}]  # verde
                    # "Se ocupacao do disco maior que\n90%, barra em vermelho."
                    # "Atualiza status CANAL3"
                    n504 = Unbundle By Name(w1101) -> ("Frames done"=w1096:u32, "connection"=→"Channel 3" →"setupCH3":bool, "conf runing"=w1100:bool, "UsedDisk"=w1082:u16, "operational"=w1087:bool)
                    "Exposures Done ch3" <- w1096
                    "Disk Storage ch3" <- w1082
                    n505 = Number To Decimal String(number=w1096) -> (decimal integer string=w1097:string)  [unwired: 1 in]
                    n506 = Greater?(x=w1082, y=u16 90) -> (0:w1093:bool)
                    n507 = Select(t=u32 16711680, s=w1093, f=u32 16860) -> (s? t:f=w1090:u32)
                    n508 = Concatenate Strings("#Exposures Done ", w1097) -> (w1095:string)
                    n509 = property on="setupCH3" class="Bool (strict)"("Blinking"=w1100) -> ()  [unwired: 2 in, 2 out]
                    n510 = property on="Disk Storage ch3" class="Slide (strict)"("Fill Color"=w1090) -> ()  [unwired: 2 in, 2 out]
                    n511 = Select(t=w1088, s=w1087, f=w1089) -> (s? t:f=w1086:cluster{u32, u32}[])
                    n512 = property on="Exposures Done ch3" class="Slide (strict)"("Caption.Text"=w1095) -> ()  [unwired: 2 in, 2 out]
                    n513 = property on="Channel 3" class="Bool (strict)"("Colors [4]"=w1086) -> ()  [unwired: 2 in, 2 out]
